vi "MIDI-Message_Parser.vi"(8 "Error In":errorcluster, 11 "MIDI Message Cluster In":T1={"Message Name"="", "Meta value"=0, "Datastring"="", "Datatype"=enum."Pause"}) -> (0 "Error Out":errorcluster, 3 "MIDI Message Cluster Out":T1={"Message Name"="", "Meta value"=0, "Datastring"="", "Datatype"=enum."Pause"})   [LabVIEW 2019]
uses:
  Controls/MIDI-Message_Cluster.ctl
  Controls/Meta_Commands.ctl
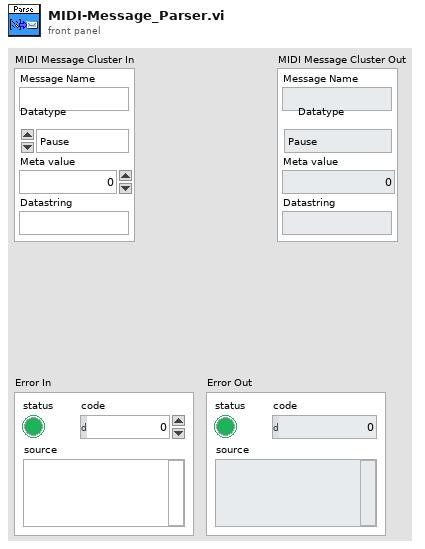
[diagram p1: front panel]
types:
  T1 = typedef "MIDI-Message_Cluster.ctl" = cluster{"Message Name":string, "Meta value":i32, "Datastring":string, "Datatype":T2}
  T2 = typedef "Meta_Commands.ctl" = enum16{"No Data", "Pause", "Loop", "Wait for Rx", "Delay", "Break", "MIDI"}
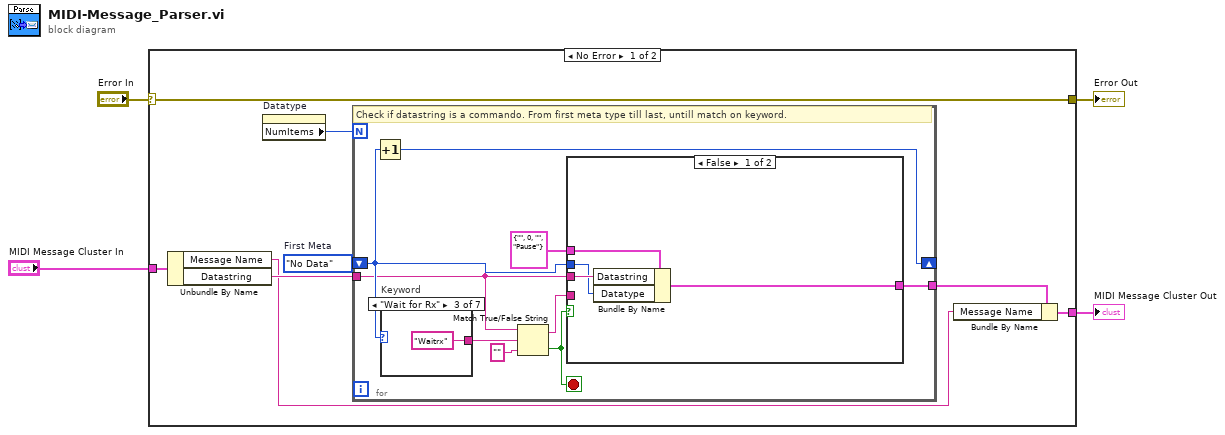
[diagram p0: block diagram]
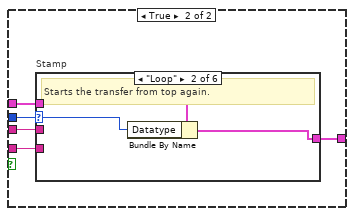
[diagram p2: hidden frame]
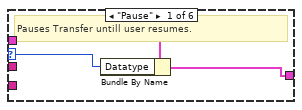
[diagram p3: hidden frame]
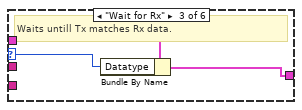
[diagram p4: hidden frame]
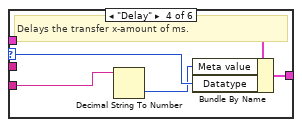
[diagram p5: hidden frame]
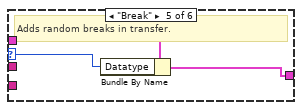
[diagram p6: hidden frame]
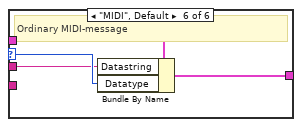
[diagram p7: hidden frame]
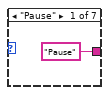
[diagram p8: hidden frame]
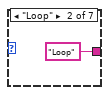
[diagram p9: hidden frame]
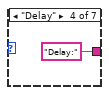
[diagram p10: hidden frame]
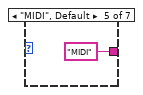
[diagram p11: hidden frame]
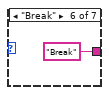
[diagram p12: hidden frame]
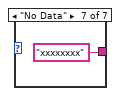
[diagram p13: hidden frame]
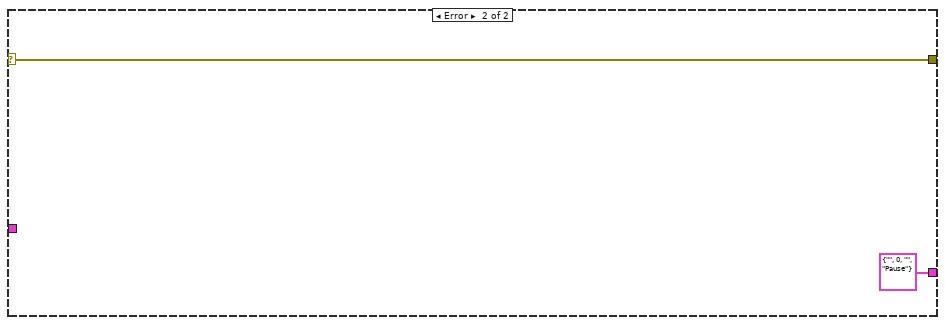
[diagram p14: hidden frame]
diagram:
  n1 = case shown="No Error" "Error In" {
    selector: "Error In" -> [w11 w59]
    tunnel: [w6 T1 {"Message Name"="", "Meta value"=0, "Datastring"="", "Datatype"=enum."Pause"} ("MIDI Message Cluster")] -> w4
    tunnel: [w11 w59] -> w3
    tunnel: "MIDI Message Cluster In" -> [w9 _]
    frame No Error {
      w12 = Meta_Commands."No Data"  # First Meta
      n2 = Unbundle By Name(w9) -> ("Message Name"=w7:string, "Datastring"=w10:string)
      n3 = property on="Datatype" class="Enum (strict)"() -> ("NumItems"=w5:u32)  [unwired: 2 in, 2 out]
      n4 = for {
        N: w5 -> [_]
        shift-right: [w13] -> _
        shift-left: w12 -> [w19]
        tunnel: w10 -> [w15]
        tunnel: [w17] -> w8
        stop <- w14 stop-if-true
        # "Check if datastring is a commando. From first meta type till last, untill match on keyword."
        n5 = Increment(x=w19) -> (x+1=w13:T2)
        n6 = case "Keyword" shown="\"Wait for Rx\"" w19 {
          tunnel: ["Pause" ("true string") "Loop" ("true string") "Waitrx" ("true string") "Delay:" ("true string") "MIDI" ("true string") "Break" ("true string") "xxxxxxxx" ("true string")] -> w20
          frame "Pause" {
          }
          frame "Loop" {
          }
          frame "Wait for Rx" {
          }
          frame "Delay" {
          }
          frame "MIDI", Default {
          }
          frame "Break" {
          }
          frame "No Data" {
          }
        }
        n7 = Match True/False String(2:"" ("false string"), 3:w20, 4:w15) -> (0:w14:bool, 1:w18:string)
        n8 = case shown="False" w14 {
          tunnel: w19 -> [w22 w30]
          tunnel: w18 -> [_ w29]
          tunnel: [w24 w28] -> w17
          tunnel: w15 -> [w23 w27]
          tunnel: T1 {"Message Name"="", "Meta value"=0, "Datastring"="", "Datatype"=enum."Pause"} ("MIDI Message Cluster") -> [w25 w26]
          frame False {
            n9 = Bundle By Name(cluster=w25, "Datastring"=w23, "Datatype"=w22) -> (w24:T1)
          }
          frame True {
            n10 = case "Stamp" shown="\"Loop\"" w30 {
              selector: w30 -> [w31 w34 w37 w43 w46 w50]
              tunnel: w29 -> [_ _ _ w40 _ _]
              tunnel: w26 -> [w33 w36 w38 w44 w47 w51]
              tunnel: [w32 w35 w39 w42 w45 w49] -> w28
              tunnel: w27 -> [_ _ _ _ _ w48]
              frame "Pause" {
                # "Pauses Transfer untill user resumes."
                n11 = Bundle By Name(cluster=w33, "Datatype"=w31) -> (w32:T1)
              }
              frame "Loop" {
                # "Starts the transfer from top again."
                n12 = Bundle By Name(cluster=w36, "Datatype"=w34) -> (w35:T1)
              }
              frame "Wait for Rx" {
                # "Waits untill Tx matches Rx data."
                n13 = Bundle By Name(cluster=w38, "Datatype"=w37) -> (w39:T1)
              }
              frame "Delay" {
                # "Delays the transfer x-amount of ms."
                n14 = Decimal String To Number(string=w40) -> (number=w41:i32)  [unwired: 2 in, 1 out]
                n15 = Bundle By Name(cluster=w44, "Meta value"=w41, "Datatype"=w43) -> (w42:T1)
              }
              frame "Break" {
                # "Adds random breaks in transfer."
                n16 = Bundle By Name(cluster=w47, "Datatype"=w46) -> (w45:T1)
              }
              frame "MIDI", Default {
                # "Ordinary MIDI-message"
                n17 = Bundle By Name(cluster=w51, "Datastring"=w48, "Datatype"=w50) -> (w49:T1)
              }
            }
          }
        }
      }
      n18 = Bundle By Name(cluster=w8, "Message Name"=w7) -> (w6:T1)
    }
    frame Error {
    }
  }
  "Error Out" <- w3
  "MIDI Message Cluster Out" <- w4
